vi "EnqueueDeluxeWash.vi"(8 "error in (no error)":errorcluster, 11 "Queue in":refnum<queue>) -> (0 "error out":errorcluster)   [LabVIEW 2018]
uses:
  MessageQueueData.ctl
  Command.ctl
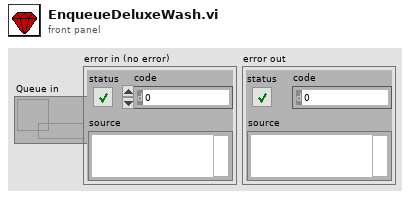
[diagram p1: front panel]
types:
  T1 = typedef "Command.ctl" = enum16{"Underbody Wash", "Soap Application", "Main High-Pressure Wash", "Clear Water Rinse", "Air Dry Cycle", "Stop"}
  T2 = typedef "MessageQueueData.ctl" = cluster{"State":T1, "Data":variant}
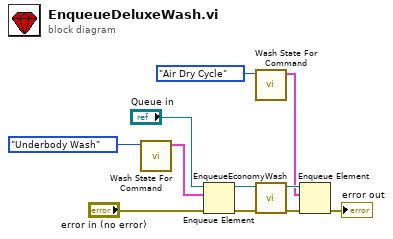
[diagram p0: block diagram]
diagram:
  n1 = call "Wash State For Command.vi"("Command"=Command."Underbody Wash") -> ("Queue Data for Command"=w3:T2)  [unwired: 10 in]
  n2 = Enqueue Element(queue="Queue in", element=w3, error in (no error)="error in (no error)") -> (queue out=w10:refnum<queue>, error out=w7:errorcluster)  [unwired: 1 in, 1 out]
  n3 = call "Wash State For Command.vi"("Command"=Command."Air Dry Cycle") -> ("Queue Data for Command"=w1:T2)  [unwired: 10 in]
  n4 = call "EnqueueEconomyWash.vi"("error in"=w7, "Queue in"=w10) -> ("error out"=w6:errorcluster, "queue out"=w9:refnum<queue>)  [unwired: 8 in]
  n5 = Enqueue Element(queue=w9, element=w1, error in (no error)=w6) -> (error out=→"error out":errorcluster)  [unwired: 1 in, 2 out]
